vi "Perform Action.vi"(8 "error in (no error)":errorcluster, 10 "Input":variant, 11 "DIO DAQmx PWM CFG in":refnum<class "DO DAQmx PWM CFG.lvclass">) -> (0 "error out":errorcluster, 2 "Output":variant, 3 "DIO DAQmx PWM CFG out":refnum<class "DO DAQmx PWM CFG.lvclass">)   [LabVIEW 2023, in "DO DAQmx PWM CFG.lvclass"]
uses:
  DO DAQmx PWM CFG.lvclass
  D:/git/HAL/HAL GOOP4/DAQmx/DAQmx Base CFG/DAQmx Base CFG.lvclass
  D:/git/HAL/HAL GOOP4/Configuration/Configuration Semaphore/CFG Semaphore.lvclass
  DAQmx/DAQmx Base CFG/DAQmx Base CFG.lvclass/DAQmx Base CFG.ctl
  Configuration/Configuration Semaphore/CFG Semaphore.lvclass/CFG Semaphore.ctl
  <vilib>/Utility/error.llb/Error Cluster From Error Code.vi
  <vilib>/ErrorRing/Error Ring.xnode
  DAQmx/DAQmx Base CFG/DAQmx Base CFG.lvclass
  <resource>/objmgr/daqmx.rc
  Configuration/Configuration Semaphore/CFG Semaphore.lvclass
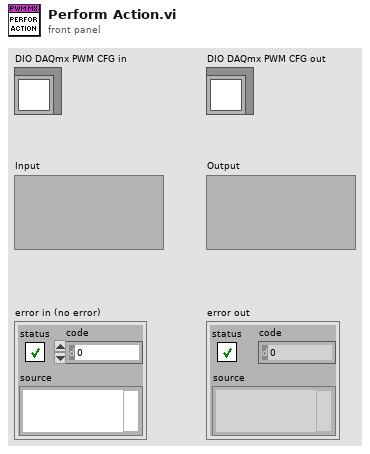
[diagram p1: front panel]
types:
  T1 = cluster{"Channel":string, "PWM Pams":cluster{"Frequency":dbl, "Duty Cycle":dbl}}
  T2 = typedef "Semaphore RefNum" = refnum<k1>
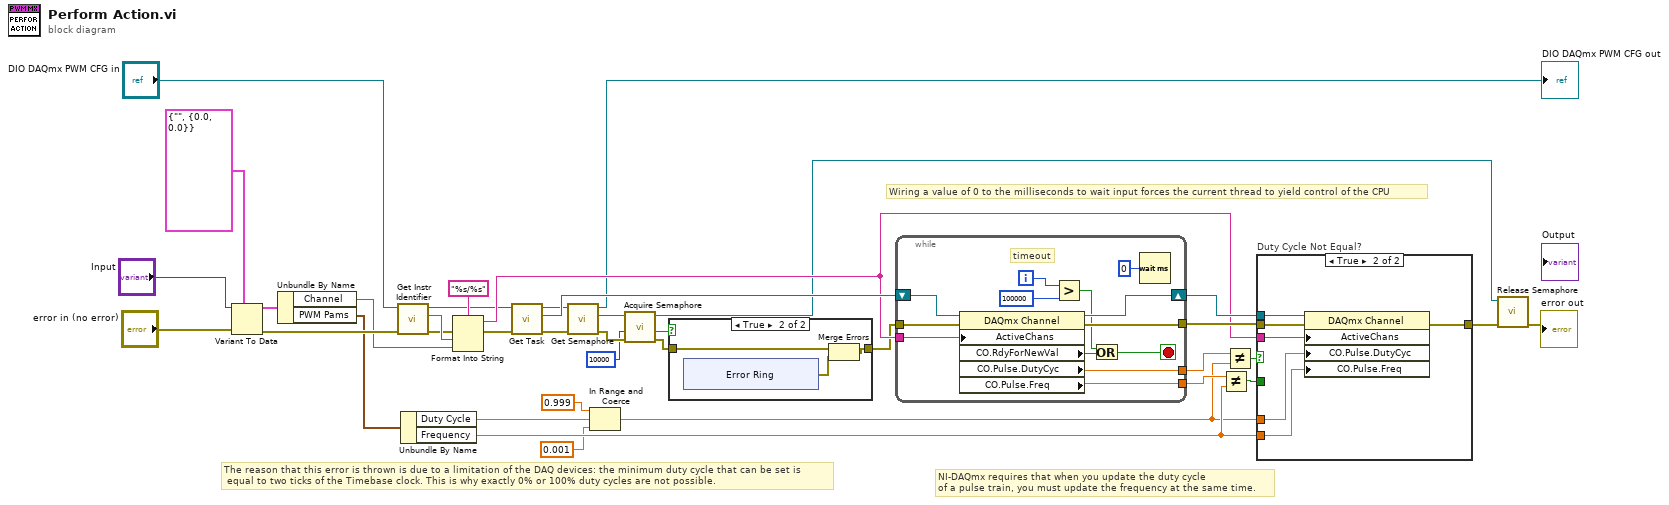
[diagram p0: block diagram]
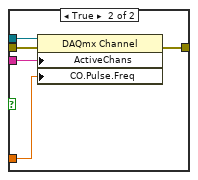
[diagram p4: hidden frame]
diagram:
  # "The reason that this error is thrown is due to a limitation of the DAQ devices: the minimum duty cycle that can be set is\n equal to two ticks of the Timebase clock. This is why exactly 0% or 100% duty cycles are not possible."
  # "Wiring a value of 0 to the milliseconds to wait input forces the current thread to yield control of the CPU"
  # "NI-DAQmx requires that when you update the duty cycle\nof a pulse train, you must update the frequency at the same time."
  n1 = Variant To Data(error in="error in (no error)", type=T1 {"Channel"="", "PWM Pams"={"Frequency"=0.0, "Duty Cycle"=0.0}}, Variant="Input") -> (data=w34:T1, error out=w35:errorcluster)
  n2 = Unbundle By Name(w34) -> ("Channel"=w29:string, "PWM Pams"=w27:cluster{"Frequency":dbl, "Duty Cycle":dbl})
  n3 = call-dynamic "Get Instr Identifier.vi"("error in (no error)"=w35, "Configuration Base in"="DIO DAQmx PWM CFG in") -> ("error out"=w28:errorcluster, "Instr Identifier"=w30:string, "Configuration Base out"=w13:refnum<class "DO DAQmx PWM CFG.lvclass">)  [unwired: 7 in]
  n4 = Unbundle By Name(w27) -> ("Duty Cycle"=w25:dbl, "Frequency"=w21:dbl)
  n5 = Format Into String(format string="%s/%s", error in=w28, w30, w29) -> (resulting string=w17:string, error out=w14:errorcluster)  [unwired: 1 in]
  n6 = call "Get Task.vi"("error in"=w14, "DAQmx Base CFG in"=w13) -> ("error out"=w15:errorcluster, "Task"=w20:refnum<k21>, "DAQmx Base CFG out"=w16:refnum<class "DO DAQmx PWM CFG.lvclass">)  [unwired: 7 in]
  n7 = call "Get Semaphore.vi"("error in (no error)"=w15, "CFG Base in"=w16) -> ("error out"=w11:errorcluster, "Semaphore"=w12:T2, "CFG Base out"=→"DIO DAQmx PWM CFG out":refnum<class "DO DAQmx PWM CFG.lvclass">)  [unwired: 7 in]
  n8 = In Range and Coerce(upper limit=0.999, x=w25, lower limit=0.001) -> (coerced(x)=w3:dbl)  [unwired: 1 out]
  n9 = call <vilib>:"Acquire Semaphore.vi"("error in (no error)"=w11, "ms timeout (-1)"=10000, "semaphore"=w12) -> ("error out"=w5:errorcluster, "timed out"=w6:bool, "semaphore out"=w9:T2)  [unwired: 2 in]
  n10 = case shown="True" w6 {
    tunnel: w5 -> [w39 w41]
    tunnel: [w39 w40] -> w4
    frame False {
    }
    frame True {
      n11 = xnode "Error Ring"() -> ("error out"=w42:errorcluster)
      n12 = Merge Errors(w41, w42) -> (w40:errorcluster)
    }
  }
  n13 = while {
    tunnel: [w59] -> w24
    tunnel: w4 -> [w58]
    tunnel: [w56] -> w19
    tunnel: w17 -> [w55]
    shift-right: [w60] -> w26
    shift-left: w20 -> [w57]
    tunnel: [w49] -> w18
    i -> [w53]
    stop <- w51 stop-if-true
    # "timeout"
    n14 = property class="DAQmx Channel"(reference=w57, error in=w58, "ActiveChans"=w55) -> (reference out=w60:refnum<k21>, error out=w49:errorcluster, "CO.RdyForNewVal"=w54:bool, "CO.Pulse.DutyCyc"=w59:dbl, "CO.Pulse.Freq"=w56:dbl)
    n15 = Greater?(x=w53, y=100000) -> (0:w48:bool)
    n16 = Or(x=w48, y=w54) -> (x .or. y?=w51:bool)
    n17 = Wait (ms)(milliseconds to wait=u32 0) -> ()  [unwired: 1 out]
  }
  n18 = Not Equal?(x=w19, y=w21) -> (x != y?=w22:bool)
  n19 = Not Equal?(x=w24, y=w3) -> (x != y?=w23:bool)
  n20 = case "Duty Cycle Not Equal?" shown="True" w23 {
    tunnel: [w63 w78] -> w32
    tunnel: w21 -> [w64 w77]
    tunnel: w18 -> [w66 w76]
    tunnel: w26 -> [w62 w75]
    tunnel: w3 -> [_ w74]
    tunnel: w22 -> [w65 _]
    tunnel: w17 -> [w61 w73]
    frame False {
      n21 = case "Frequeny Not Equal?" shown="False" w65 {
        tunnel: w66 -> [w67 w72]
        tunnel: w64 -> [_ w69]
        tunnel: [w67 w71] -> w63
        tunnel: w62 -> [_ w70]
        tunnel: w61 -> [_ w68]
        frame False {
        }
        frame True {
          n22 = property class="DAQmx Channel"(reference=w70, error in=w72, "ActiveChans"=w68, "CO.Pulse.Freq"=w69) -> (error out=w71:errorcluster)  [unwired: 1 out]
        }
      }
    }
    frame True {
      n23 = property class="DAQmx Channel"(reference=w75, error in=w76, "ActiveChans"=w73, "CO.Pulse.DutyCyc"=w74, "CO.Pulse.Freq"=w77) -> (error out=w78:errorcluster)  [unwired: 1 out]
    }
  }
  n24 = call <vilib>:"Release Semaphore.vi"("error in (no error)"=w32, "semaphore"=w9) -> ("error out"=→"error out":errorcluster)  [unwired: 4 in, 1 out]
